vi "connect_information.vi"(10 "路径":path) -> (2 "connect info":string)   [LabVIEW 2018]
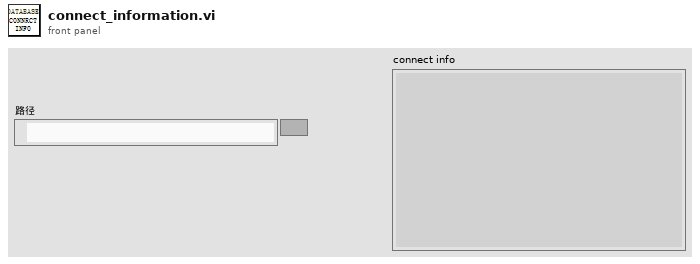
[diagram p1: front panel]
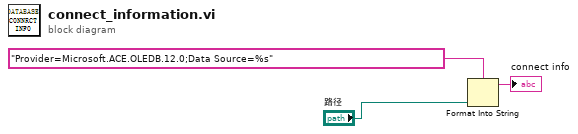
[diagram p0: block diagram]
diagram:
  n1 = Format Into String(format string="Provider=Microsoft.ACE.OLEDB.12.0;Data Source=%s" ("格式字符串"), "路径") -> (resulting string=→"connect info":string)  [unwired: 2 in, 1 out]
